vi "Ring_creator.vi"() -> ()   [LabVIEW 2014]
uses:
  <vilib>/myRIO/Instrument Drivers/Onboard IO/AudioOut Block/typedefs/AudioOut Block Reference.ctl
  <vilib>/myRIO/Common/Instrument Driver Framework/Utilities/typedefs/myRIO Generic Hardware Reference.ctl
  <vilib>/myRIO/Common/Instrument Driver Framework/Utilities/typedefs/Hardware Version Enum.ctl
  <vilib>/myRIO/Common/Instrument Driver Framework/Utilities/typedefs/myRIO v1.0 Reference.ctl
  <vilib>/myRIO/Common/Instrument Driver Framework/Utilities/typedefs/Generic FPGA Reference.ctl
  <vilib>/myRIO/Common/Instrument Driver Framework/myRIO v1.0/AudioOut Block/typedefs/AudioOut Block Channels List.ctl
  <vilib>/myRIO/Common/Instrument Driver Framework/myRIO v1.0/AudioOut Block/typedefs/AudioOut Block Channels Enum.ctl
  <vilib>/myRIO/Common/Instrument Driver Framework/Utilities/typedefs/Analog Scaling Constants.ctl
  <vilib>/userdefined/High Color/nirio_resource_hc.ctl
  <vilib>/myRIO/Common/Instrument Driver Framework/Utilities/vis/Is FPGA Ref Available.vi
  <vilib>/myRIO/Common/Instrument Driver Framework/myRIO v1.0/AudioOut Block/vis/myRIO v1.1 Open Throughput AudioOut (N Samples).vi
  <vilib>/myRIO/Instrument Drivers/Onboard IO/AudioOut Block/vis/Write.vi
  <vilib>/myRIO/Common/Instrument Driver Framework/Utilities/vis/Validate Channels.vi
  <vilib>/Utility/VariantDataType/GetNumericInfo.vi
  <vilib>/Utility/error.llb/Error Cluster From Error Code.vi
  <vilib>/myRIO/Common/Instrument Driver Framework/myRIO v1.0/myRIO v1.1 Open Throughput.vi
  <vilib>/myRIO/Common/Instrument Driver Framework/myRIO v1.0/AudioOut Block/vis/myRIO v1.0 Get Scaling Constants AudioOut Block.vi
  <vilib>/myRIO/Common/Instrument Driver Framework/myRIO v1.0/AudioOut Block/vis/myRIO v1.0 Reserve AudioOut Block.vi
  <vilib>/myRIO/Common/Instrument Driver Framework/myRIO v1.0/Resource Manager/vis/myRIO v1.0 Open Writing DMA.vi
  <vilib>/myRIO/Common/Instrument Driver Framework/myRIO v1.0/myRIO v1.0 Close.vi
  <vilib>/myRIO/Common/Instrument Driver Framework/myRIO v1.0/AudioOut Block/vis/myRIO v1.0 AudioOut Block Write.vi
  <vilib>/myRIO/Express VI/Onboard IO/AudioOut/AudioOut Express VI.xnode
  <vilib>/myRIO/Instrument Drivers/Onboard IO/AudioOut Block/vis/myRIO AudioOut N Samples Open.xnode
  <vilib>/myRIO/Instrument Drivers/Onboard IO/AudioOut Block/AudioOut Block.lvlib
panel:
  out "Waveform Graph":dbl[](graph)
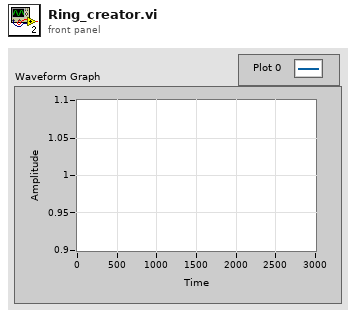
[diagram p1: front panel]
types:
  T1 = typedef "AudioOut Block.lvlib/AudioOut Block Reference.ctl" = cluster{"myRIO Reference":T2, "AudioOut (N Samples) Channels List":T6, "AudioOut (N Samples) Scaling Constants List":T8[]}
  T2 = typedef "myRIO Generic Hardware Reference.ctl" = cluster{"myRIO Model":T3, "myRIO Hardware Reference":T4}
  T3 = typedef "Hardware Version Enum.ctl" = enum16{"Unknown", "myRIO-1900", "myRIO-1950"}
  T4 = typedef "myRIO v1.0 Reference.ctl" = cluster{"Generic FPGA Reference":T5, "Allow multiple opens":bool}
  T5 = typedef "Generic FPGA Reference.ctl" = refnum<k20>
  T6 = typedef "AudioOut Block Channels List.ctl" = T7[]
  T7 = typedef "AudioOut Block Channels Enum.ctl" = enum16{"Not Connected", "AudioOut/Left (N Samples)", "AudioOut/Right (N Samples)"}
  T8 = typedef "Analog Scaling Constants.ctl" = cluster{"LSB Weight (Volts)":dbl, "Offset (Volts)":dbl, "Signed?":bool}
  T9 = typedef "nirio_resource_hc.ctl" = tag
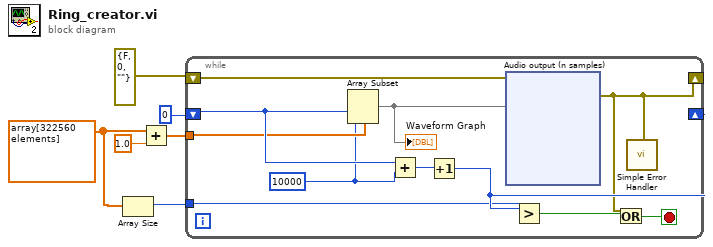
[diagram p0: block diagram]
diagram:
  w1 = dbl[] array[322560 elements] ("Y")
  n1 = Array Size(array=w1) -> (size(s)=w4:i32)
  n2 = Add(x=w1, y=1.0) -> (x+y=w5:dbl[])
  n3 = while {
    tunnel: w5 -> [w11]
    tunnel: w4 -> [w14]
    shift-right: [w16] -> _
    shift-left: 0 ("index") -> [w17]
    shift-right: [w9] -> _
    shift-left: errorcluster {"status"=FALSE, "code"=0, "source"=""} ("error in (no error)") -> [w10]
    stop <- w12 stop-if-true
    w8 = 10000 ("length")
    n4 = Array Subset(array=w11, index=w17, length=w8) -> (w7:dbl[])
    "Waveform Graph" <- w7
    n5 = Add(x=w17, y=w8) -> (x+y=w15:i32)
    n6 = Increment(x=w15) -> (x+1=w16:i32)
    n7 = xnode "Audio output (n samples)"("AudioOut/Left (N Samples)"=w7, "AudioOut/Right (N Samples)"=w7, "error in (no error)"=w10) -> ("error out"=w9:errorcluster)
    n8 = Greater?(x=w16, y=w14) -> (0:w13:bool)
    n9 = Or(x=w9, y=w13) -> (x .or. y?=w12:bool)
    n10 = call <vilib>:"Simple Error Handler.vi"("error in (no error)"=w9) -> ()  [unwired: 4 in, 5 out]
  }
